vi "SP Delete Marker from Table.vi"(7 "CH Control In":T1={"Trace Orientation"=enum."Overlay", "Frequency"={"Change Frequency"=FALSE, "Start"=500.0, "Stop"=1500.0, "Units"=enum."MHz"}, "Markers"=[], "Traces"=[]} {"Traces"."Reference" format="%#.2g"; "Traces"."Display Data" items=["Data", "Memory", "Data/Memory"]; "Traces"."Format" items=["Log Mag", "Phase", "Expanded Phase", "Delay", "Smith", "Polar", "Lin Mag", "SWR", "Loss", "Real", "Imaginary"]; "Traces"."Scale" min=0.001 step=1.0 format="%#.2g"; "Traces"."Position" min=0.0 max=10.0; "Frequency"."Stop" format="%.3g"; "Frequency"."Start" format="%.3g"}, 8 "error in (no error)":errorcluster, 10 "Marker Table Ref":refnum<vi>) -> (0 "error out":errorcluster, 1 "Deleted Marker":i8, 2 "Marker Table Ref":refnum<vi>, 5 "CH Control Out":T1={"Trace Orientation"=enum."Overlay", "Frequency"={"Change Frequency"=FALSE, "Start"=500.0, "Stop"=1500.0, "Units"=enum."MHz"}, "Markers"=[], "Traces"=[]} {"Traces"."Reference" format="%#.2g"; "Traces"."Display Data" items=["Data", "Memory", "Data/Memory"]; "Traces"."Format" items=["Log Mag", "Phase", "Expanded Phase", "Delay", "Smith", "Polar", "Lin Mag", "SWR", "Loss", "Real", "Imaginary"]; "Traces"."Scale" min=0.001 step=1.0 format="%#.2g"; "Traces"."Position" min=0.0 max=10.0; "Frequency"."Stop" format="%.3g"; "Frequency"."Start" format="%.3g"})   [LabVIEW 2011]
uses:
  TypeDefs/SP Display Plot Controls Cluster.ctl
  TypeDefs/SP Frequency Units.ctl
  TypeDefs/SP Marker Cluster.ctl
  TypeDefs/SP Marker Type.ctl
  TypeDefs/SP Display Trace Controls.ctl
  TypeDefs/SP Display Format.ctl
  TypeDefs/SP Display Data.ctl
panel:
  # "Div"
  # "Div"
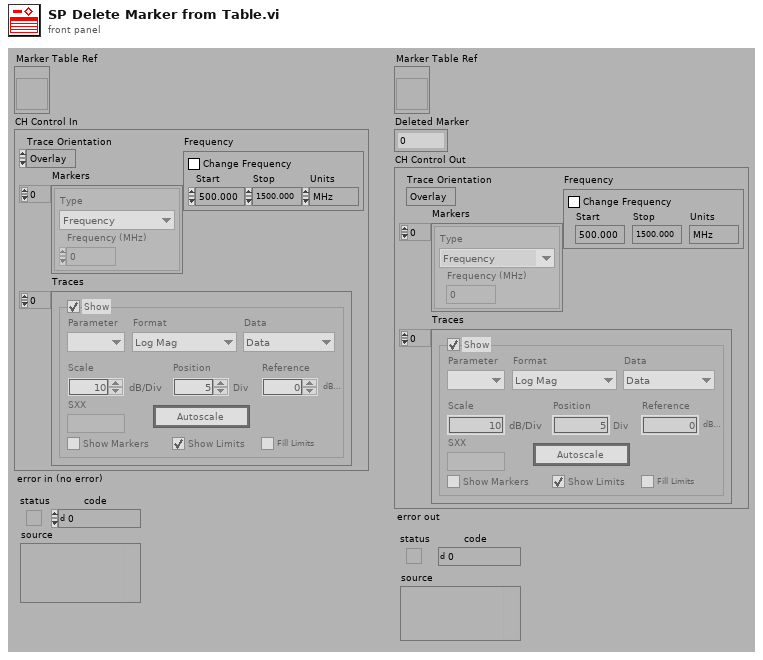
[diagram p1: front panel]
types:
  T1 = typedef "SP Display Plot Controls Cluster.ctl" = cluster{"Trace Orientation":enum32{"Overlay", "Split"}, "Frequency":cluster{"Change Frequency":bool, "Start":dbl, "Stop":dbl, "Units":T2}, "Markers":T3[], "Traces":T5[]}
  T2 = typedef "SP Frequency Units.ctl" = enum16{"Hz", "kHz", "MHz", "GHz", "Points"}
  T3 = typedef "SP Marker Cluster.ctl" = cluster{"Type":T4, "Frequency (MHz)":dbl}
  T4 = typedef "SP Marker Type.ctl" = enum16{"Frequency", "Trace Maximum", "Trace Minimum", "Limit Maximum", "Limit Minimum"}
  T5 = typedef "SP Display Trace Controls.ctl" = cluster{"Trace On":bool, "Measure":i32, "Format":T6, "Autoscale":bool, "Reference":dbl, "\nRefUnit":string, "Position":dbl, "Scale":dbl, "ScaleUnit":string, "LimitOn":bool, "LimitFill":bool, "Display Data":T7, "Show Markers":bool, "SXX":string}
  T6 = typedef "SP Display Format.ctl" = i32
  T7 = typedef "SP Display Data.ctl" = u16
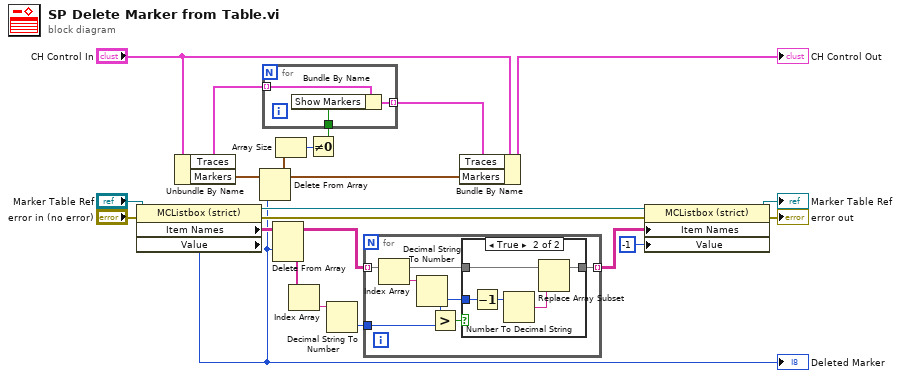
[diagram p0: block diagram]
diagram:
  n1 = property class="MCListbox (strict)"(reference="Marker Table Ref", error in="error in (no error)") -> (reference out=w18:refnum<vi>, error out=w19:errorcluster, "Item Names"=w17:string[][], "Value"=w7:i32)
  "Deleted Marker" <- w7
  n2 = Unbundle By Name("CH Control In") -> ("Traces"=w3:T5[], "Markers"=w8:T3[])
  n3 = Delete From Array(array=w8, index=w7) -> (array with subset deleted=w5:T3[])  [unwired: 1 in, 1 out]
  n4 = Delete From Array(array=w17, index (row)=w7) -> (deleted portion=w16:string[], array with subset deleted=w13:string[][])  [unwired: 2 in]
  n5 = Array Size(array=w5) -> (size(s)=w4:i32)
  n6 = Index Array(array=w16) -> (element=w15:string)  [unwired: 1 in]
  n7 = Not Equal To 0?(x=w4) -> (x != 0?=w2:bool)
  n8 = for {
    tunnel: w3 -> [w24] mode=indexing
    tunnel: w2 -> [w25]
    tunnel: [w23] -> w1 mode=indexing
    n9 = Bundle By Name(cluster=w24, "Show Markers"=w25) -> (w23:T5)
  }
  n10 = Decimal String To Number(string=w15) -> (number=w14:i32)  [unwired: 3 out]
  n11 = for {
    tunnel: w13 -> [w28] mode=indexing
    tunnel: w14 -> [w30]
    tunnel: [w26] -> w12 mode=indexing
    n12 = Index Array(array=w28) -> (element=w31:string)  [unwired: 1 in]
    n13 = Decimal String To Number(string=w31) -> (number=w27:i32)  [unwired: 3 out]
    n14 = Greater?(x=w27, y=w30) -> (0:w29:bool)
    n15 = case shown="True" w29 {
      tunnel: w28 -> [w32 w35]
      tunnel: w27 -> [_ w37]
      tunnel: [w32 w33] -> w26
      frame False {
      }
      frame True {
        n16 = Decrement(x=w37) -> (x-1=w36:i32)
        n17 = Number To Decimal String(number=w36) -> (decimal integer string=w34:string)  [unwired: 1 out]
        n18 = Replace Array Subset(array=w35, new element=w34) -> (w33:string[])  [unwired: 1 in]
      }
    }
  }
  n19 = Bundle By Name(cluster="CH Control In", "Traces"=w1, "Markers"=w5) -> (→"CH Control Out":T1)
  n20 = property class="MCListbox (strict)"(reference=w18, error in=w19, "Item Names"=w12, "Value"=-1 ("Value (Signaling)")) -> (reference out=→"Marker Table Ref":refnum<vi>, error out=→"error out":errorcluster)
